vi "GetInputTerminalControlRef.vi"(9 "Input Terminal Name":string, 10 "Algorithm VI Path":path, 11 "Application in":refnum<vi>) -> (2 "vi reference":refnum<vi>, 3 "Control out":refnum<vi>)   [LabVIEW 2021]
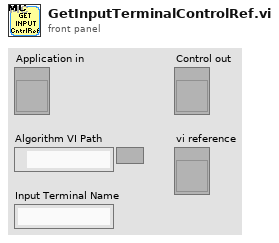
[diagram p1: front panel]
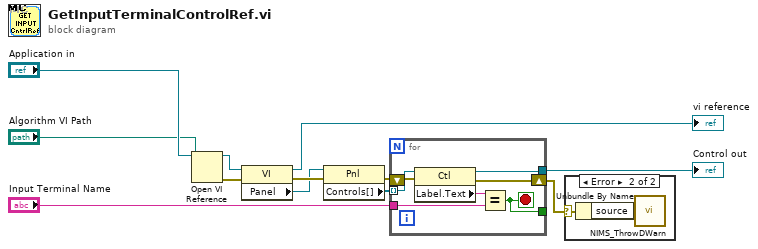
[diagram p0: block diagram]
diagram:
  n1 = Open VI Reference(application reference (local)="Application in", vi path="Algorithm VI Path") -> (vi reference=w3:refnum<vi>, error out=w4:errorcluster)  [unwired: 4 in]
  n2 = property class="VI"(reference=w3, error in=w4) -> (reference out=→"vi reference":refnum<vi>, error out=w6:errorcluster, "Panel"=w5:refnum<vi>)
  n3 = property class="Pnl"(reference=w5, error in=w6) -> (error out=w8:errorcluster, "Controls[]"=w7:refnum<vi>[])  [unwired: 1 out]
  n4 = for {
    tunnel: w7 -> [w18] mode=indexing
    tunnel: "Input Terminal Name" -> [w16]
    tunnel: [w15] -> w10
    tunnel: [w14] -> _
    shift-right: [w13] -> w11
    shift-left: w8 -> [w19]
    stop <- w14 stop-if-true
    n5 = property class="Ctl"(reference=w18, error in=w19) -> (reference out=w15:refnum<vi>, error out=w13:errorcluster, "Label.Text"=w17:string)
    n6 = Equal?(x=w17, y=w16) -> (x = y?=w14:bool)
  }
  "Control out" <- w10
  n7 = case shown="Error" w11 {
    selector: w11 -> [_ w21]
    frame No Error {
    }
    frame Error {
      n8 = Unbundle By Name(w21) -> ("source"=w20:string)
      n9 = call <vilib>:"NIMS_ThrowDWarn.vi"("DWarn"=w20) -> ()  [unwired: 1 in]
    }
  }
